vi "host_burst_search.vi"(4 "m":u64=3, 5 "L":u64=20, 6 "T":u64=10958, 7 "ph_times":u64[](array[numeric])) -> (0 "width":u64[](array[numeric]), 1 "size":u64[](array[numeric]), 2 "i_start":u64[](array[numeric]), 3 "burst_start":u64[](array[numeric]))   [LabVIEW 2009]
panel:
  out "current ph. \narrival time":u64
  out "i":u64
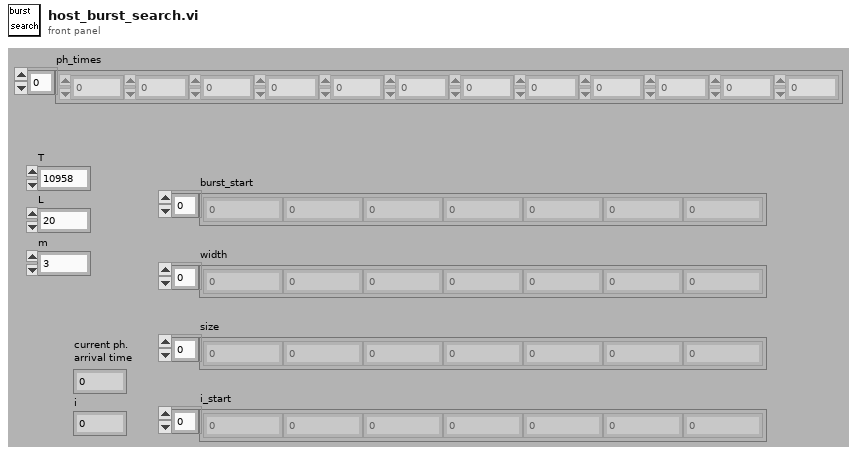
[diagram p1: front panel]
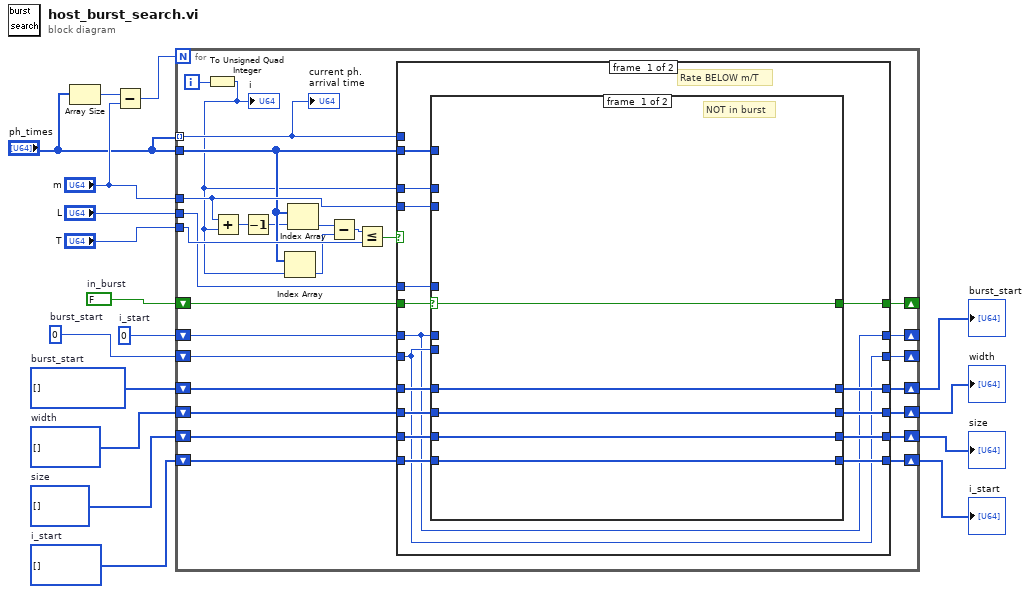
[diagram p0: block diagram]
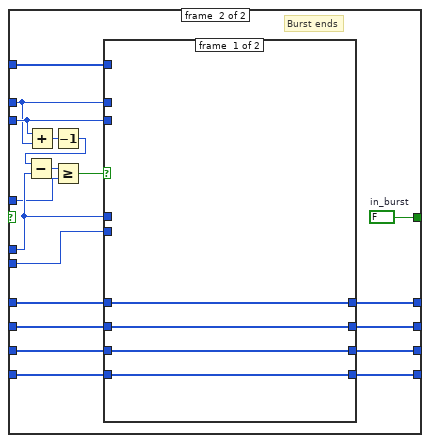
[diagram p2: hidden frame]
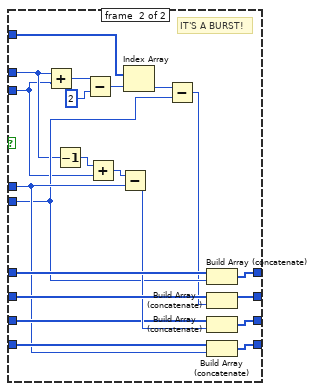
[diagram p3: hidden frame]
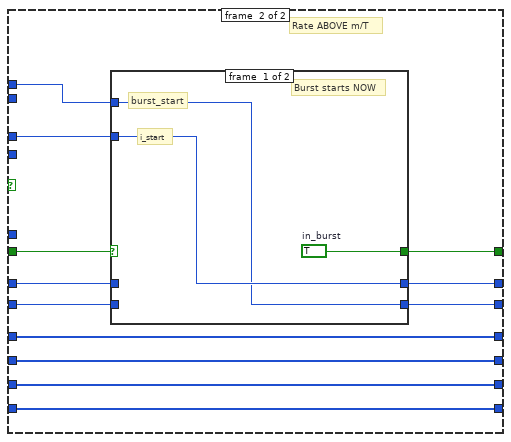
[diagram p4: hidden frame]
diagram:
  w2 = u64 0  # i_start
  w8 = u64[] []  # i_start
  w9 = u64[] []  # size
  w10 = u64[] []  # width
  w11 = u64[] []  # burst_start
  w3 = u64 0  # burst_start
  w12 = FALSE  # in_burst
  n1 = Array Size(array="ph_times") -> (size(s)=w15:i32)
  n2 = Subtract(x=w15, y="m") -> (x-y=w13:u64)
  n3 = for {
    N: w13 -> [_]
    tunnel: "m" -> [w30]
    tunnel: "L" -> [w25]
    tunnel: "T" -> [w42]
    shift-right: [w39] -> _
    shift-left: w12 -> [w41]
    shift-right: [w37] -> _
    shift-left: w2 -> [w38]
    shift-right: [w35] -> _
    shift-left: w3 -> [w36]
    shift-right: [w27] -> w1
    shift-left: w9 -> [w32]
    shift-right: [w26] -> w4
    shift-left: w8 -> [w33]
    shift-right: [w28] -> w5
    shift-left: w10 -> [w31]
    shift-right: [w29] -> w7
    shift-left: w11 -> [w34]
    tunnel: "ph_times" -> [w24]
    tunnel: "ph_times" -> [w20] mode=indexing
    i -> [w18]
    n4 = To Unsigned Quad Integer(1:w18) -> (0:w19:u64)
    "i" <- w19
    n5 = Add(x=w30, y=w19) -> (x+y=w44:u64)
    n6 = Decrement(x=w44) -> (x-1=w23:u64)
    n7 = Index Array(array=w24, index=w19) -> (element=w21:u64)
    n8 = Index Array(array=w24, index=w23) -> (element=w22:u64)
    n9 = Subtract(x=w22, y=w21) -> (x-y=w43:u64)
    n10 = Less Or Equal?(x=w43, y=w42) -> (x <= y?=w40:bool)
    n11 = case shown="False" w40 {
      tunnel: w41 -> [w49 w120]
      tunnel: w19 -> [w55 w121]
      tunnel: [w60 w119] -> w39
      tunnel: w38 -> [w46 w112]
      tunnel: [w46 w118] -> w37
      tunnel: w36 -> [w47 w111]
      tunnel: [w47 w117] -> w35
      tunnel: w34 -> [w56 w116]
      tunnel: w33 -> [w59 w113]
      tunnel: w32 -> [w58 w114]
      tunnel: w31 -> [w57 w115]
      tunnel: w30 -> [w54 _]
      tunnel: [w53 w116] -> w29
      tunnel: [w52 w115] -> w28
      tunnel: [w51 w114] -> w27
      tunnel: [w50 w113] -> w26
      tunnel: w25 -> [w48 _]
      tunnel: w24 -> [w45 _]
      tunnel: w20 -> [_ w110]
      frame #0 {
        # "Rate BELOW m/T"
        n12 = case shown="True" w49 {
          selector: w49 -> [w65 _]
          tunnel: [w65 w67] -> w60
          tunnel: w46 -> [_ w72]
          tunnel: w47 -> [_ w76]
          tunnel: w59 -> [w61 w81]
          tunnel: w58 -> [w62 w82]
          tunnel: w57 -> [w63 w84]
          tunnel: w56 -> [w64 w83]
          tunnel: w55 -> [_ w74]
          tunnel: w54 -> [_ w75]
          tunnel: [w64 w80] -> w53
          tunnel: [w63 w79] -> w52
          tunnel: [w62 w78] -> w51
          tunnel: [w61 w77] -> w50
          tunnel: w48 -> [_ w69]
          tunnel: w45 -> [_ w66]
          frame #0 {
            # "NOT in burst"
          }
          frame #1 {
            w67 = FALSE  # in_burst
            # "Burst ends"
            n13 = Add(x=w75, y=w74) -> (x+y=w73:u64)
            n14 = Decrement(x=w73) -> (x-1=w71:u64)
            n15 = Subtract(x=w71, y=w72) -> (x-y=w70:u64)
            n16 = Greater Or Equal?(x=w70, y=w69) -> (x >= y?=w68:bool)
            n17 = case shown="True" w68 {
              tunnel: w84 -> [w87 w109]
              tunnel: w83 -> [w88 w107]
              tunnel: w82 -> [w86 w102]
              tunnel: w81 -> [w85 w101]
              tunnel: w72 -> [_ w100]
              tunnel: [w88 w99] -> w80
              tunnel: [w87 w98] -> w79
              tunnel: [w86 w97] -> w78
              tunnel: [w85 w96] -> w77
              tunnel: w76 -> [_ w95]
              tunnel: w74 -> [_ w93]
              tunnel: w75 -> [_ w92]
              tunnel: w66 -> [_ w91]
              frame #0 {
              }
              frame #1 {
                # "IT'S A BURST!"
                n18 = Add(x=w93, y=w92) -> (x+y=w94:u64)
                n19 = Decrement(x=w93) -> (x-1=w105:u64)
                n20 = Subtract(x=w94, y=u64 2) -> (x-y=w108:u64)
                n21 = Add(x=w105, y=w92) -> (x+y=w104:u64)
                n22 = Subtract(x=w104, y=w100) -> (x-y=w103:u64)
                n23 = Index Array(array=w91, index=w108) -> (element=w90:u64)
                n24 = Subtract(x=w90, y=w95) -> (x-y=w89:u64)
                n25 = Build Array (concatenate)(w107, w95) -> (w99:u64[])
                n26 = Build Array (concatenate)(w109, w89) -> (w98:u64[])
                n27 = Build Array (concatenate)(w102, w103) -> (w97:u64[])
                n28 = Build Array (concatenate)(w101, w100) -> (w96:u64[])
              }
            }
          }
        }
      }
      frame #1 {
        # "Rate ABOVE m/T"
        n29 = case shown="False" w120 {
          selector: w120 -> [_ w127]
          tunnel: w121 -> [w124 _]
          tunnel: [w123 w127] -> w119
          tunnel: [w124 w126] -> w118
          tunnel: [w122 w125] -> w117
          tunnel: w112 -> [_ w126]
          tunnel: w111 -> [_ w125]
          tunnel: w110 -> [w122 _]
          frame #0 {
            w123 = TRUE  # in_burst
            # "burst_start"
            # "i_start"
            # "Burst starts NOW"
          }
          frame #1 {
            # "Burst already started"
          }
        }
      }
    }
    "current ph. \narrival time" <- w20
  }
  "burst_start" <- w7
  "size" <- w1
  "i_start" <- w4
  "width" <- w5
